vi "generate array.vi"(8 "error in":errorcluster, 10 "tag bus configurable plugin module configuration":refnum<class "PID Module configuration.lvclass">, 11 "array":T1) -> (0 "error out":errorcluster)   [LabVIEW 2014, in "PID Module editor node.lvclass"]
uses:
  PID Module editor node.lvclass
  PID array reference.ctl
  PID array element.ctl
  module/configuration/PID Module configuration.lvclass
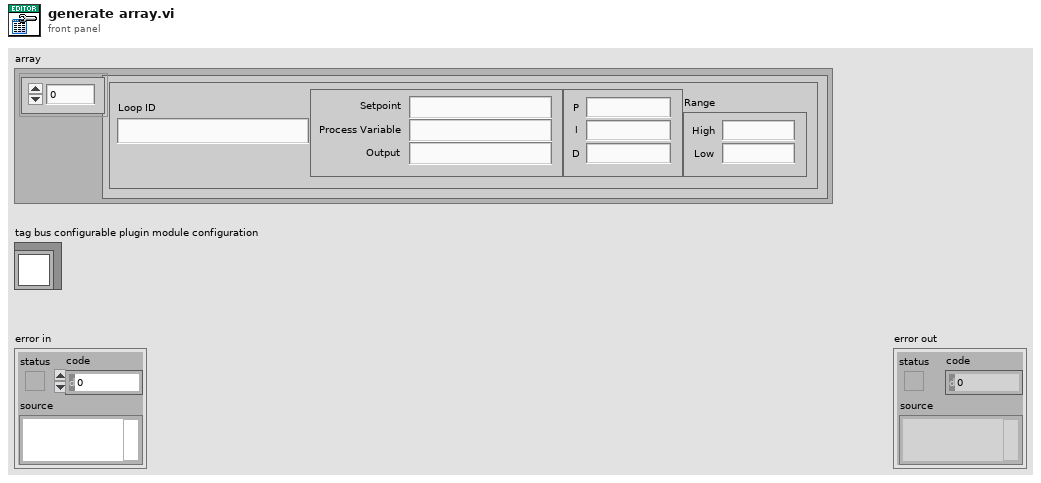
[diagram p1: front panel]
types:
  T1 = typedef "PID Module editor node.lvclass/PID array reference.ctl" = refnum<vi>
  T2 = typedef "PID Module editor node.lvclass/PID array element.ctl" = cluster{"Loop ID":string, "Tags":cluster{"Setpoint":string, "Process Variable":string, "Output":string}, "Gains":cluster{"P":dbl, "I":dbl, "D":dbl}, "Range":cluster{"High":dbl, "Low":dbl}}
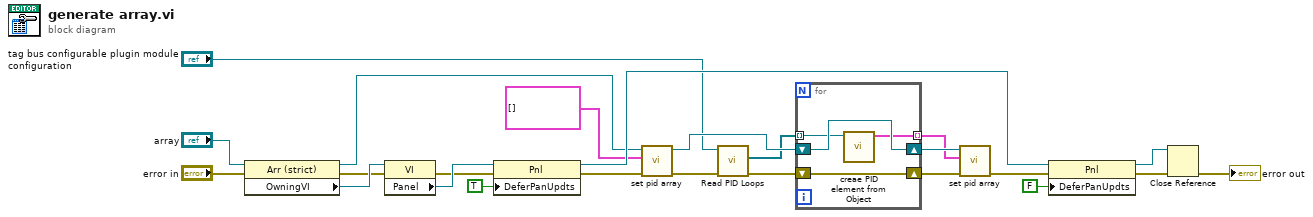
[diagram p0: block diagram]
diagram:
  n1 = property class="Arr (strict)"(reference="array", error in="error in") -> (reference out=w12:T1, error out=w15:errorcluster, "OwningVI"=w16:refnum<vi>)
  n2 = property class="VI"(reference=w16, error in=w15) -> (error out=w21:errorcluster, "Panel"=w22:refnum<vi>)  [unwired: 1 out]
  n3 = property class="Pnl"(reference=w22, error in=w21, "DeferPanUpdts"=TRUE ("Defer Panel Updates")) -> (reference out=w19:refnum<vi>, error out=w11:errorcluster)
  n4 = call "set pid array.vi"("error in (no error)"=w11, "Array"=T2[] [], "Array in"=w12) -> ("error out"=w3:errorcluster, "Array out"=w9:T1)  [unwired: 7 in]
  n5 = call-dynamic "Read PID Loops.vi"("error in (no error)"=w3, "Tagbus PID Module configuration in"="tag bus configurable plugin module configuration") -> ("error out"=w2:errorcluster, "PID Loops"=w1:refnum<class "PID Loop.lvclass">[])  [unwired: 7 in, 1 out]
  n6 = for {
    shift-right: [w25] -> w7
    shift-left: w2 -> [w25]
    shift-right: [w28] -> w8
    shift-left: w9 -> [w28]
    tunnel: w1 -> [w27] mode=indexing
    tunnel: [w26] -> w6 mode=indexing
    n7 = call "creae PID element from Object.vi"("PID Loop in"=w27) -> ("line"=w26:T2)  [unwired: 10 in]
  }
  n8 = call "set pid array.vi"("error in (no error)"=w7, "Array"=w6, "Array in"=w8) -> ("error out"=w5:errorcluster)  [unwired: 7 in, 1 out]
  n9 = property class="Pnl"(reference=w19, error in=w5, "DeferPanUpdts"=FALSE ("Defer Panel Updates")) -> (reference out=w13:refnum<vi>, error out=w18:errorcluster)
  n10 = Close Reference(reference=w13, error in (no error)=w18) -> (error out=→"error out":errorcluster)
